vi "_GetLensValues.vi"(3 "RampingParams":u8[](array[numeric]), 4 "Lens List":u8[](array[numeric]), 5 "Lenses":T1[](array[typedef])) -> (1 "UserValues":string[](array[string]), 2 "LensesOut":T1[](array[typedef]))   [LabVIEW 2015]
uses:
  Type/_Lens Property.ctl
  Type/_Log Command.ctl
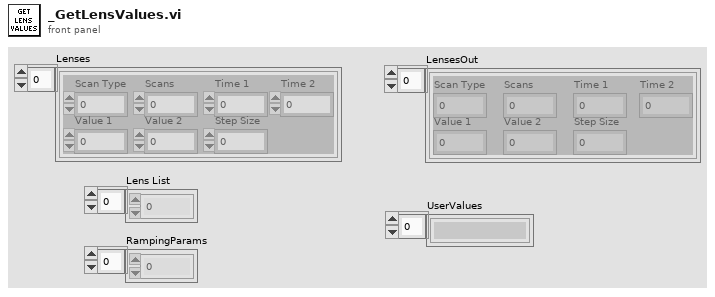
[diagram p1: front panel]
types:
  T1 = typedef "_Lens Property.ctl" = cluster{"Scan Type":u8, "Scans":i32, "Time 1":dbl, "Time 2":dbl, "Value 1":dbl, "Value 2":dbl, "Step Size":dbl}
  T2 = typedef "_Log Command.ctl" = enum16{"No Command", "Open", "Read", "Write", "Close", "Check Size"}
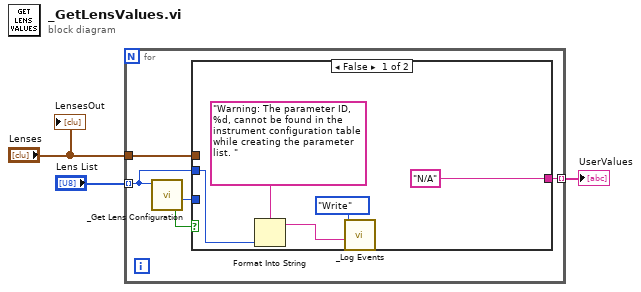
[diagram p0: block diagram]
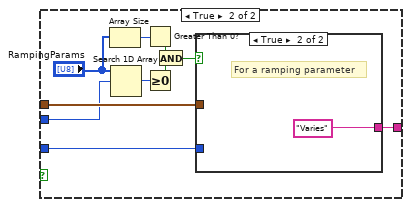
[diagram p2: hidden frame]
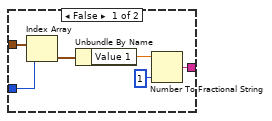
[diagram p3: hidden frame]
diagram:
  n1 = for {
    tunnel: "Lenses" -> [w8]
    tunnel: "Lens List" -> [w4] mode=indexing
    tunnel: [w6] -> w2 mode=indexing
    n2 = call "_Get Lens Configuration.vi"("Channel #"=w4) -> ("Found"=w5:bool, "Config Row#"=w7:i32)  [unwired: 1 in, 4 out]
    n3 = case shown="False" w5 {
      tunnel: w8 -> [_ w23]
      tunnel: w7 -> [_ w22]
      tunnel: ["N/A" w21] -> w6
      tunnel: w4 -> [w12 w20]
      frame False {
        n4 = Format Into String(format string="Warning: The parameter ID, %d, cannot be found in the instrument configuration table while creating the parameter list. ", w12) -> (resulting string=w11:string)  [unwired: 2 in, 1 out]
        n5 = call "_Log Events.vi"("Event"=w11, "Log Command"=_Log_Command."Write") -> ()  [unwired: 6 in, 2 out]
      }
      frame True {
        n6 = Array Size(array="RampingParams") -> (size(s)=w17:i32)
        n7 = Search 1D Array(1D array="RampingParams", element=w20) -> (index of element=w19:i32)  [unwired: 1 in]
        n8 = Greater Than 0?(x=w17) -> (x > 0?=w15:bool)
        n9 = Greater Or Equal To 0?(x=w19) -> (x >= 0?=w16:bool)
        n10 = And(x=w15, y=w16) -> (x .and. y?=w14:bool)
        n11 = case shown="True" w14 {
          tunnel: w23 -> [w29 _]
          tunnel: w22 -> [w28 _]
          tunnel: [w24 "Varies"] -> w21
          frame False {
            n12 = Index Array(array=w29, index=w28) -> (element=w25:T1)
            n13 = Unbundle By Name(w25) -> ("Value 1"=w27:dbl)
            n14 = Number To Fractional String(number=w27, precision (6)=i16 1) -> (F-format string=w24:string)  [unwired: 2 out]
          }
          frame True {
            # "For a ramping parameter"
          }
        }
      }
    }
  }
  "UserValues" <- w2
  "LensesOut" <- "Lenses"
